vi "Maui.Config.Locate.vi"(6 "Create?":bool, 8 "error in (no error)":errorcluster, 9 "Path":path, 10 "Application Name":string, 11 "Maui.Config in":refnum<class "Maui.Config.lvclass">) -> (0 "error out":errorcluster, 1 "Exists?":bool, 2 "Path":path, 3 "Maui.Config out":refnum<class "Maui.Config.lvclass">, 4 "Created?":bool)   [LabVIEW 2019, in "Maui.Config.lvclass"]
uses:
  Maui.Config.lvclass
panel:
  in  "Variant":variant
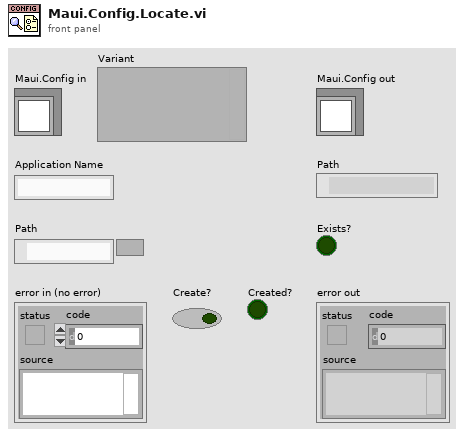
[diagram p1: front panel]
types:
  T1 = enum16{"open", "replace", "create", "open or create", "replace or create", "replace or create with confirmation"}
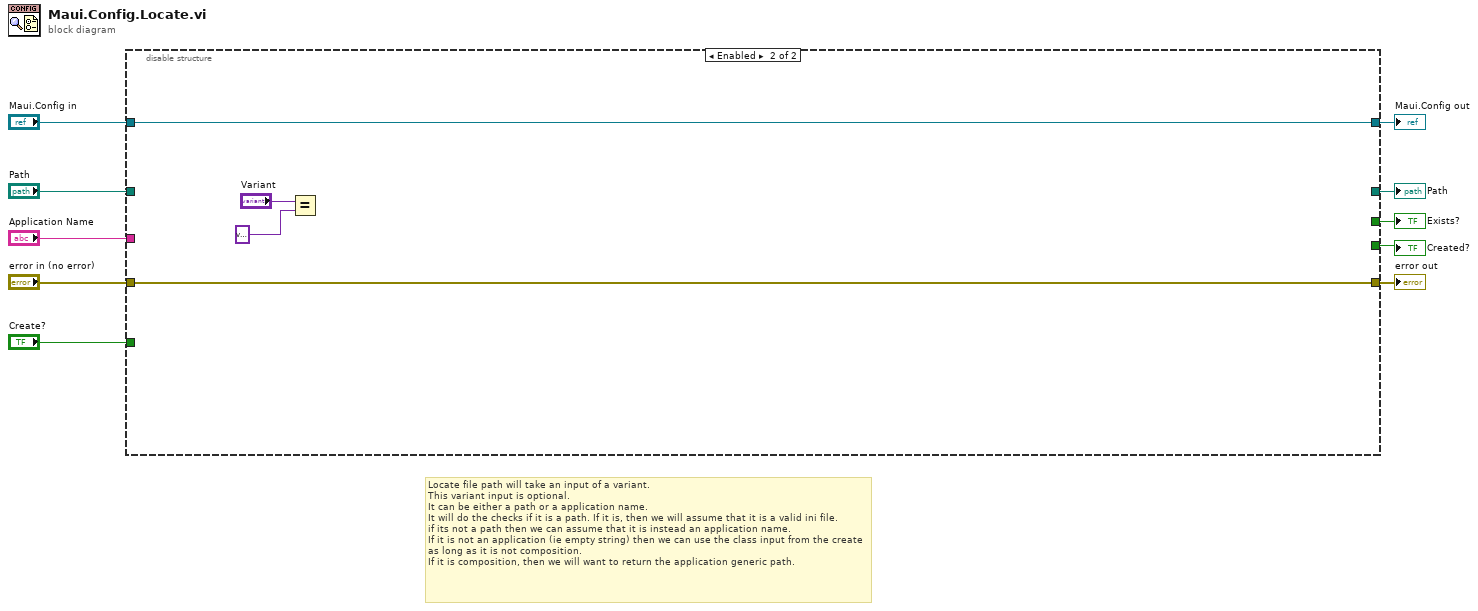
[diagram p0: block diagram]
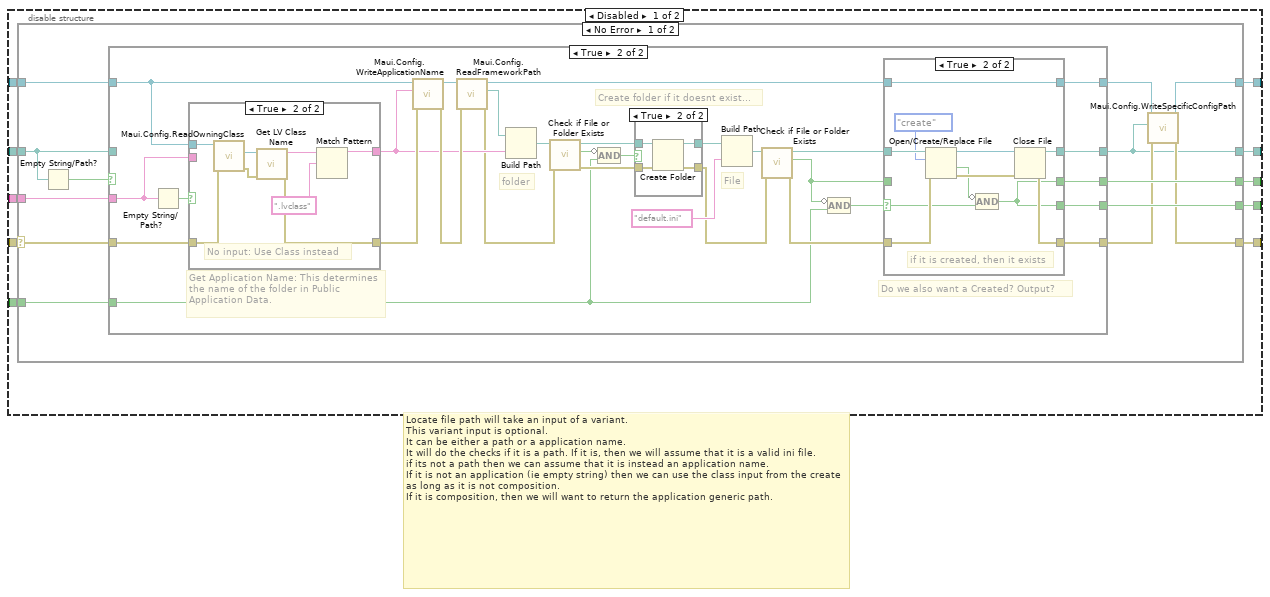
[diagram p2: hidden frame]
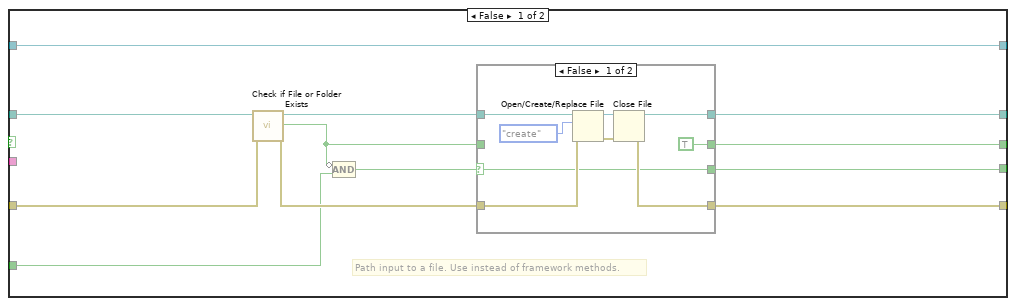
[diagram p3: hidden frame]
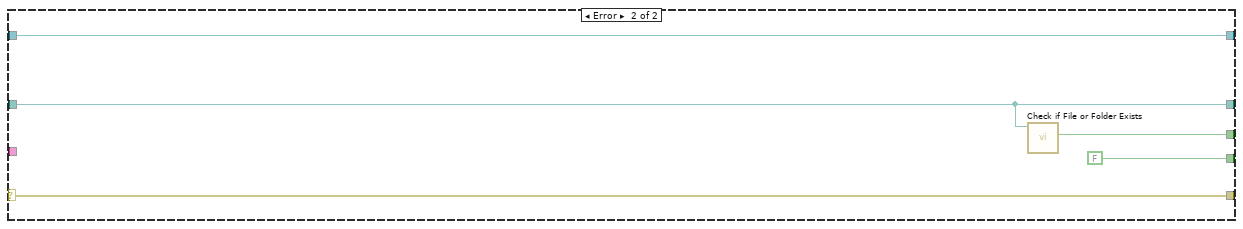
[diagram p8: hidden frame]
diagram:
  # "Locate file path will take an input of a variant.\nThis variant input is optional. \nIt can be either a path or a application name.\nIt will do the checks if it is a path. If it is, then we will assume that it is a valid ini file.\nif its not a path then we can assume that it is instead an application name.\nIf it is not an application (ie empty string) then we can use the class input from the create as long as it is not composition.\nIf it is composition, then we will want to return the application generic path."
  n1 = disable-structure shown="Enabled" {
    disable-tunnel: "error in (no error)" -> [w20 w128]
    disable-tunnel: [w19 w128] -> w9
    disable-tunnel: "Maui.Config in" -> [w18 w129]
    disable-tunnel: [w17 w129] -> w7
    disable-tunnel: "Application Name" -> [w16 _]
    disable-tunnel: "Path" -> [w15 _]
    disable-tunnel: "Create?" -> [w14 _]
    disable-tunnel: [w13 _] -> w3
    disable-tunnel: [w12 _] -> w2
    disable-tunnel: [w11 _] -> w1
    frame Disabled {
      # "Locate file path will take an input of a variant.\nThis variant input is optional. \nIt can be either a path or a application name.\nIt will do the checks if it is a path. If it is, then we will assume that it is a valid ini file.\nif its not a path then we can assume that it is instead an application name.\nIf it is not an application (ie empty string) then we can use the class input from the create as long as it is not composition.\nIf it is composition, then we will want to return the application generic path."
      n2 = case shown="No Error" w20 {
        selector: w20 -> [w33 w123]
        tunnel: [w23 w123] -> w19
        tunnel: [w25 w125] -> w17
        tunnel: w18 -> [w31 w125]
        tunnel: w16 -> [w32 _]
        tunnel: w15 -> [w21 w122]
        tunnel: w14 -> [w29 _]
        tunnel: [w28 w121] -> w13
        tunnel: [w27 FALSE] -> w12
        tunnel: [w22 w122] -> w11
        frame No Error {
          n3 = Empty String/Path?(string/path=w21) -> (empty?=w30:bool)
          n4 = case shown="True" w30 {
            tunnel: w32 -> [_ w83]
            tunnel: [w45 w77] -> w26
            tunnel: w31 -> [w45 w81]
            tunnel: [w42 w86] -> w24
            tunnel: w33 -> [w43 w87]
            tunnel: w29 -> [w37 w60]
            tunnel: [w39 w70] -> w22
            tunnel: [w36 w69] -> w28
            tunnel: [w34 w68] -> w27
            tunnel: w21 -> [w44 _]
            frame False {
              # "Path input to a file. Use instead of framework methods."
              n5 = call <vilib>:"Check if File or Folder Exists.vi"("error in (no error)"=w43, "path"=w44) -> ("error out"=w41:errorcluster, "file or folder exists?"=w35:bool, "dup path"=w40:path)  [unwired: 7 in]
              n6 = Compound Arithmetic op=AND(invert w35, w37) -> (w38:bool)
              n7 = case shown="False" w38 {
                selector: w38 -> [w46 w55]
                tunnel: [w48 w58] -> w42
                tunnel: w41 -> [w51 w58]
                tunnel: w40 -> [w49 w57]
                tunnel: [w50 w57] -> w39
                tunnel: [TRUE w56] -> w36
                tunnel: w35 -> [_ w56]
                tunnel: [w46 w55] -> w34
                frame False {
                  n8 = Open/Create/Replace File(file path (use dialog)=w49, error in=w51, operation (0:open)=T1."create") -> (refnum out=w53:refnum<file>, error out=w52:errorcluster)  [unwired: 3 in, 1 out]
                  n9 = Close File(refnum=w53, error in=w52) -> (path=w50:path, error out=w48:errorcluster)
                }
                frame True {
                }
              }
            }
            frame True {
              # "Create folder if it doesnt exist..."
              # "Do we also want a Created? Output?"
              # "File"
              # "Get Application Name: This determines the name of the folder in Public Application Data."
              # "folder"
              n10 = Empty String/Path?(string/path=w83) -> (empty?=w82:bool)
              n11 = case shown="True" w82 {
                tunnel: w81 -> [_ w117]
                tunnel: w87 -> [w112 w119]
                tunnel: [w111 w113] -> w78
                tunnel: w83 -> [w111 _]
                tunnel: [w112 w118] -> w88
                frame False {
                  # "Use input instead of class"
                }
                frame True {
                  # "No input: Use Class instead"
                  n12 = call "Maui.Config.ReadOwningClass.vi"("error in (no error)"=w119, "Maui.Config in"=w117) -> ("error out"=w120:errorcluster, "Owning Class"=w116:refnum<class>)  [unwired: 7 in, 1 out]
                  n13 = call <vilib>:"Get LV Class Name.vi"("error in (no error)"=w120, "object"=w116) -> ("error out"=w118:errorcluster, "class name"=w115:string)  [unwired: 8 in]
                  n14 = Match Pattern(string=w115, regular expression=".lvclass") -> (before substring=w113:string)  [unwired: 1 in, 3 out]
                }
              }
              n15 = call "Maui.Config.WriteApplicationName.vi"("error in (no error)"=w88, "Application Name"=w78, "Maui.Config in"=w81) -> ("error out"=w84:errorcluster, "Maui.Config out"=w80:refnum<class "Maui.Config.lvclass">)  [unwired: 7 in]
              n16 = call "Maui.Config.ReadFrameworkPath.vi"("error in (no error)"=w84, "Maui.Config in"=w80) -> ("error out"=w64:errorcluster, "Framework Path"=w79:path, "Maui.Config out"=w76:refnum<class "Maui.Config.lvclass">)  [unwired: 7 in]
              n17 = Build Path(base path=w79, name or relative path=w78) -> (appended path=w67:path)
              n18 = call <vilib>:"Check if File or Folder Exists.vi"("error in (no error)"=w64, "path"=w67) -> ("error out"=w65:errorcluster, "file or folder exists?"=w61:bool, "dup path"=w66:path)  [unwired: 7 in]
              n19 = Compound Arithmetic op=AND(invert w61, w60) -> (w59:bool)
              n20 = case shown="True" w59 {
                tunnel: w66 -> [w90 w94]
                tunnel: w65 -> [w89 w93]
                tunnel: [w89 w92] -> w63
                tunnel: [w90 w91] -> w62
                frame False {
                }
                frame True {
                  n21 = Create Folder(path (use dialog)=w94, error in=w93) -> (created path=w91:path, error out=w92:errorcluster)  [unwired: 1 in, 1 out]
                }
              }
              n22 = Build Path(base path=w62, name or relative path="default.ini") -> (appended path=w71:path)
              n23 = call <vilib>:"Check if File or Folder Exists.vi"("error in (no error)"=w63, "path"=w71) -> ("error out"=w85:errorcluster, "file or folder exists?"=w73:bool, "dup path"=w75:path)  [unwired: 7 in]
              n24 = Compound Arithmetic op=AND(invert w73, w60) -> (w74:bool)
              n25 = case shown="True" w74 {
                selector: w74 -> [w95 w101]
                tunnel: [w98 w110] -> w77
                tunnel: w76 -> [w98 w110]
                tunnel: [w99 w104] -> w86
                tunnel: w85 -> [w99 w105]
                tunnel: w75 -> [w96 w109]
                tunnel: w73 -> [w97 _]
                tunnel: [w96 w103] -> w70
                tunnel: [w97 w100] -> w69
                tunnel: [w95 w100] -> w68
                frame False {
                }
                frame True {
                  # "if it is created, then it exists"
                  n26 = Open/Create/Replace File(file path (use dialog)=w109, error in=w105, operation (0:open)=T1."create") -> (refnum out=w107:refnum<file>, cancelled=w102:bool, error out=w106:errorcluster)  [unwired: 3 in]
                  n27 = Compound Arithmetic op=AND(invert w102, w101) -> (w100:bool)
                  n28 = Close File(refnum=w107, error in=w106) -> (path=w103:path, error out=w104:errorcluster)
                }
              }
            }
          }
          n29 = call "Maui.Config.WriteSpecificConfigPath.vi"("error in (no error)"=w24, "Specific Configuration"=w22, "Maui.Config in"=w26) -> ("error out"=w23:errorcluster, "Maui.Config out"=w25:refnum<class "Maui.Config.lvclass">)  [unwired: 7 in]
        }
        frame Error {
          n30 = call <vilib>:"Check if File or Folder Exists.vi"("path"=w122) -> ("file or folder exists?"=w121:bool)  [unwired: 8 in, 2 out]
        }
      }
    }
    frame Enabled {
      n31 = Equal?(x="Variant", y=variant) -> ()  [unwired: 1 out]
    }
  }
  "error out" <- w9
  "Maui.Config out" <- w7
  "Exists?" <- w3
  "Created?" <- w2
  "Path" <- w1
